vi "emi_Create Error.vi"(1 "Error Code":i32(ring) items=["0 No Error"=0, "1 Invalid input parameter"=1, "6 Generic file IO "=6, "7 File not Found"=7, "35 Generic Pring Error"=35, "37 Device not Found"=37, "39 Device Unit Error"=39, "40 Could fot Open Device"=40, "42 Generic Error"=42, "52 Unknown Message"=52, "98 Bad File type"=98, "99 Bad File Version"=99, "100 Bad Data in File"=100, "1018 Unspecefied Error"=1018, "1041 Incorrect Password"=1041, "1043 Feature not in this version"=1043, "1109 Unsuported Data type"=1109, "1444 Did not close sucessfully"=1444], 5 "Warning instead of Error(F)":bool, 7 "Error(T)":bool=TRUE, 9 "error in (no error)":errorcluster, 12 "Create Source data (T)":bool=TRUE, 13 "Source String(\"\")":string, 14 "Append String(\"\")":string) -> (10 "error out":errorcluster)   [LabVIEW 2011]
doc: "Generates a specific custom error based on Error Code. If Error code is below 5000, 500 will be added to the code.\n\nIf Error(T) is wired, this has to be true for either error or warning to be created.\nIf Warning istead of Error is true, a warning will be created not an error, when Error(T) is true.\nIf Create Source Data(T) is false, no source data wil be generated. Making whis false will requir fewer resources.\nIf Append sting is included, this will be included int eh source infor with the <Append> tag\nThis vi normaly creates a source string like : Calling.vi -> CallersCallers.vi -> ..., If Source String is used, the source will be: \"Source String\" in Calling.vi -> CallersCallers.vi -> ...,"
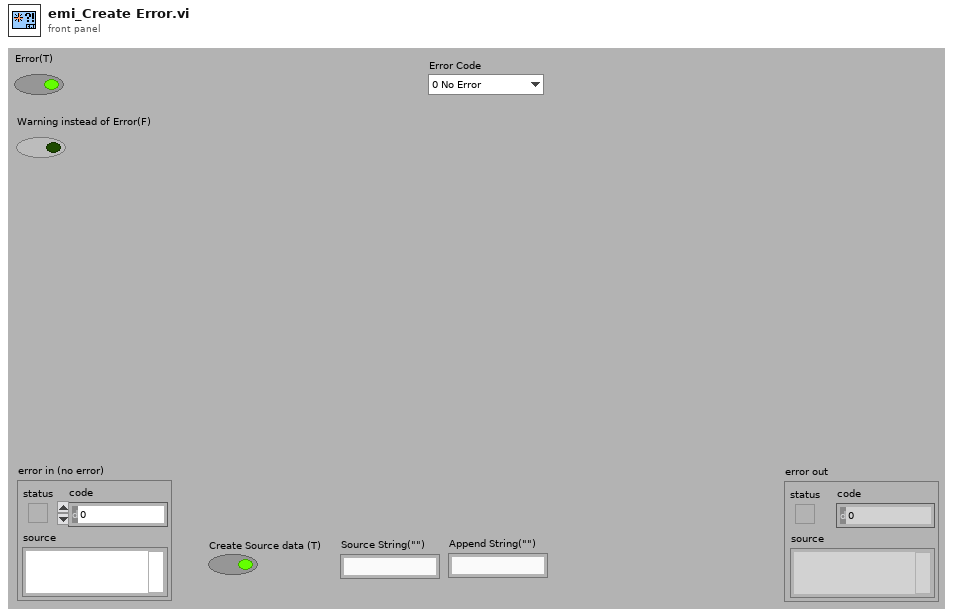
[diagram p1: front panel]
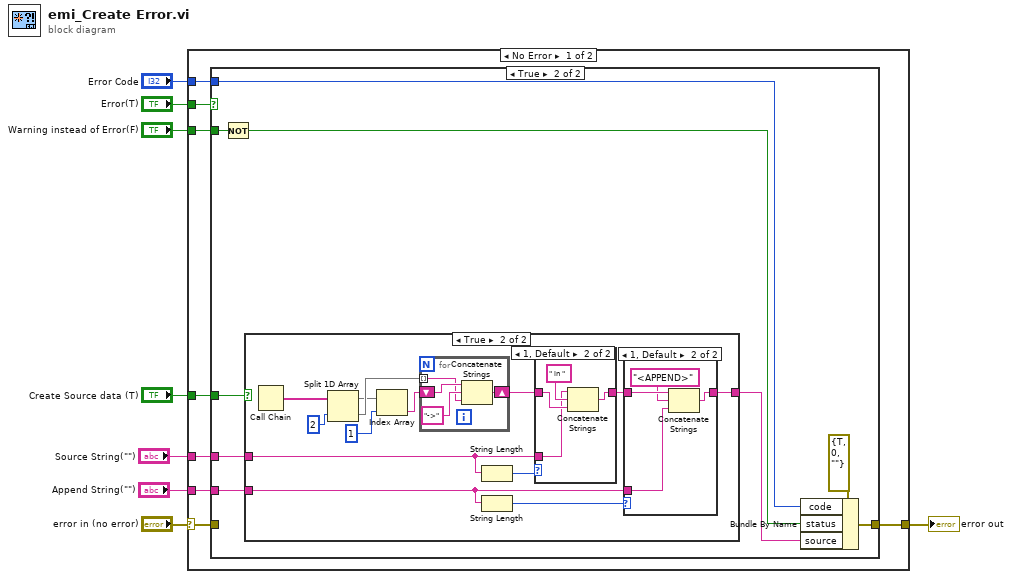
[diagram p0: block diagram]
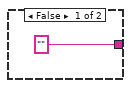
[diagram p3: hidden frame]
diagram:
  n1 = case shown="No Error" "error in (no error)" {
    selector: "error in (no error)" -> [w16 w55]
    tunnel: [w15 w55] -> w7
    tunnel: "Error Code" -> [w13 _]
    tunnel: "Error(T)" -> [w14 _]
    tunnel: "Warning instead of Error(F)" -> [w12 _]
    tunnel: "Create Source data (T)" -> [w11 _]
    tunnel: "Append String(\"\")" -> [w10 _]
    tunnel: "Source String(\"\")" -> [w9 _]
    frame No Error {
      n2 = case shown="True" w14 {
        tunnel: w16 -> [w17 _]
        tunnel: [w17 w23] -> w15
        tunnel: w13 -> [_ w22]
        tunnel: w12 -> [_ w25]
        tunnel: w11 -> [_ w20]
        tunnel: w10 -> [_ w19]
        tunnel: w9 -> [_ w18]
        frame False {
        }
        frame True {
          n3 = Not(x=w25) -> (.not. x?=w24:bool)
          n4 = case shown="True" w20 {
            tunnel: ["" w38] -> w21
            tunnel: w19 -> [_ w39]
            tunnel: w18 -> [_ w31]
            frame False {
            }
            frame True {
              n5 = Call Chain() -> (call chain=w28:string[])
              n6 = Split 1D Array(array=w28, index=2) -> (first subarray=w34:string[], second subarray=w36:string[])
              n7 = Index Array(array=w34, index=1) -> (element=w35:string)
              n8 = for {
                tunnel: w36 -> [w46] mode=indexing
                shift-right: [w49] -> w29
                shift-left: w35 -> [w47]
                n9 = Concatenate Strings(w47, "->" ("string"), w46) -> (w49:string)
              }
              n10 = String Length(string=w31) -> (length=w32:i32)
              n11 = String Length(string=w39) -> (length=w40:i32)
              n12 = case shown="1, Default" w32 {
                tunnel: w31 -> [_ w43]
                tunnel: [w41 w42] -> w30
                tunnel: w29 -> [w41 w45]
                frame 0 {
                }
                frame 1, Default {
                  n13 = Concatenate Strings(w43, " in " ("string"), w45) -> (w42:string)
                }
              }
              n14 = case shown="1, Default" w40 {
                tunnel: w39 -> [_ w51]
                tunnel: [w50 w54] -> w38
                tunnel: w30 -> [w50 w53]
                frame 0 {
                  # "No append info"
                }
                frame 1, Default {
                  n15 = Concatenate Strings(w53, "<APPEND>", w51) -> (w54:string)
                }
              }
            }
          }
          n16 = Bundle By Name(cluster=errorcluster {"status"=TRUE, "code"=0, "source"=""} ("error IO"), "code"=w22, "status"=w24, "source"=w21) -> (w23:errorcluster)
        }
      }
    }
    frame Error {
    }
  }
  "error out" <- w7
